vi "Flatten Packet To Message String.vi"(8 "error in (no error)":errorcluster, 10 "Message Packet":variant, 11 "IMessagingProtocol in":refnum<class "IMessagingProtocol.lvclass">) -> (0 "error out":errorcluster, 3 "Packet as Message String":string)   [LabVIEW 2019, in "Network Interface.lvlib" / "IMessagingProtocol.lvclass"]
uses:
  <vilib>/gpm_packages/@cs/Network-Sink/Source/Network Interface/IMessagingProtocol/IMessagingProtocol.lvclass
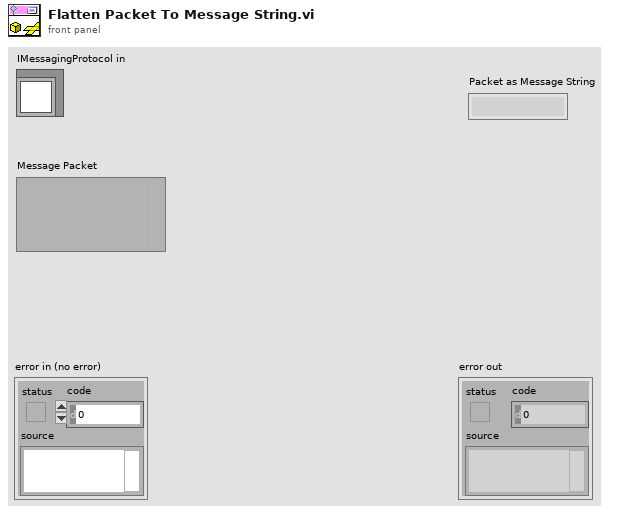
[diagram p1: front panel]
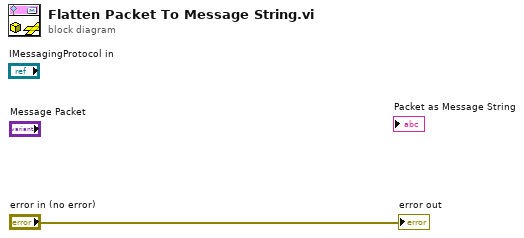
[diagram p0: block diagram]
diagram:
  "error out" <- "error in (no error)"
